vi "Actor Core.vi"(8 "error in":errorcluster, 11 "Air Cooler Application":refnum<class "Air Cooler Application.lvclass">) -> (0 "error out":errorcluster, 3 "Actor out":refnum<class "Actor.lvclass">)   [LabVIEW 2025, in "Air Cooler Application.lvlib" / "Air Cooler Application.lvclass"]
doc: "This is Actor Core.vi, the main message handling loop for Actors. An actor usually just sits in this loop and processes messages as they arrive. Any error returned by the message Do.vi call will stop the loop, with error code 43 as the canonical signal to stop with no error sent to caller. Descendants may override that in Handle Error.vi."
uses:
  Air Cooler Application.lvclass
  C:/Program Files/National Instruments/LabVIEW 2025/vi.lib/ActorFramework/Actor/Actor.lvclass
  <vilib>/ActorFramework/Actor/Actor.lvclass
  Cooler/Cooler/Cooler.lvclass
  Live User Controller/Live User Controller.lvclass
  C:/Program Files/National Instruments/LabVIEW 2025/ProjectTemplates/Source/Core/Feedback Evaporative Cooler/Cooler Controller/Cooler Controller/Cooler Controller.lvclass
  <vilib>/ActorFramework/Actor/Actor.lvclass/Actor.ctl
  <vilib>/ActorFramework/Message Enqueuer/Message Enqueuer.lvclass/Message Enqueuer.ctl
  Air Cooler Application.lvclass/Air Cooler Application.ctl
  <vilib>/ActorFramework/Stop Msg/Stop Msg.lvclass/Stop Msg.ctl
  Programmatic Controller/Programmatic Controller.lvclass
  Swap Controllers Msg/Swap Controllers Msg.lvclass/Swap Controllers Msg.ctl
  Cooler Controller/Write Cooler Enqueuer Msg/Write Cooler Enqueuer Msg.lvclass/Write Cooler Enqueuer Msg.ctl
  Cooler/Write Controller Enqueuer Msg/Write Controller Enqueuer Msg.lvclass/Write Controller Enqueuer Msg.ctl
  <vilib>/ActorFramework/Message Enqueuer/Init from Existing Queue.vi
  <vilib>/ActorFramework/Message Enqueuer/Enqueue.vi
  <vilib>/ActorFramework/Message Enqueuer/Enqueue Critical.vi
  Cooler Controller/Write Cooler Enqueuer Msg/Write Cooler Enqueuer Msg.lvclass
  C:/Program Files/National Instruments/LabVIEW 2025/vi.lib/ActorFramework/Message/Message.lvclass
  Cooler/Write Controller Enqueuer Msg/Write Controller Enqueuer Msg.lvclass
  <vilib>/ActorFramework/Stop Msg/Stop Msg.lvclass
  Swap Controllers Msg/Swap Controllers Msg.lvclass
  <vilib>/ActorFramework/Message Priority Queue/Priority Enqueue.vi
  <vilib>/ActorFramework/Message Enqueuer/Message Enqueuer.lvclass
panel:
  in  "DNL_Controller Selection":enum32{"UI Option 1", "UI Option 2"}(radio)
  in  "Stop":bool
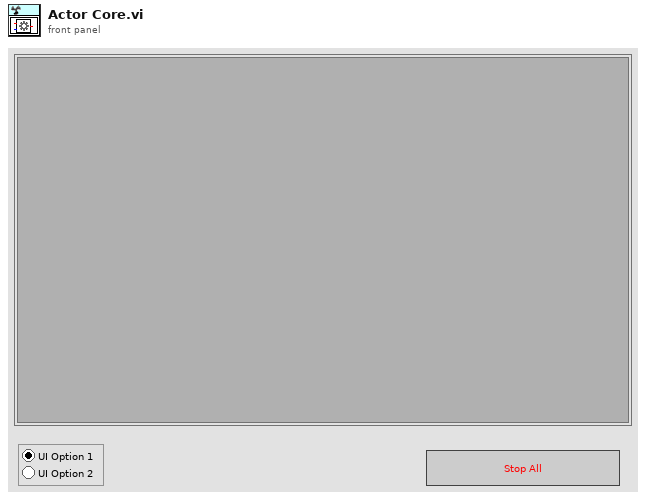
[diagram p1: front panel]
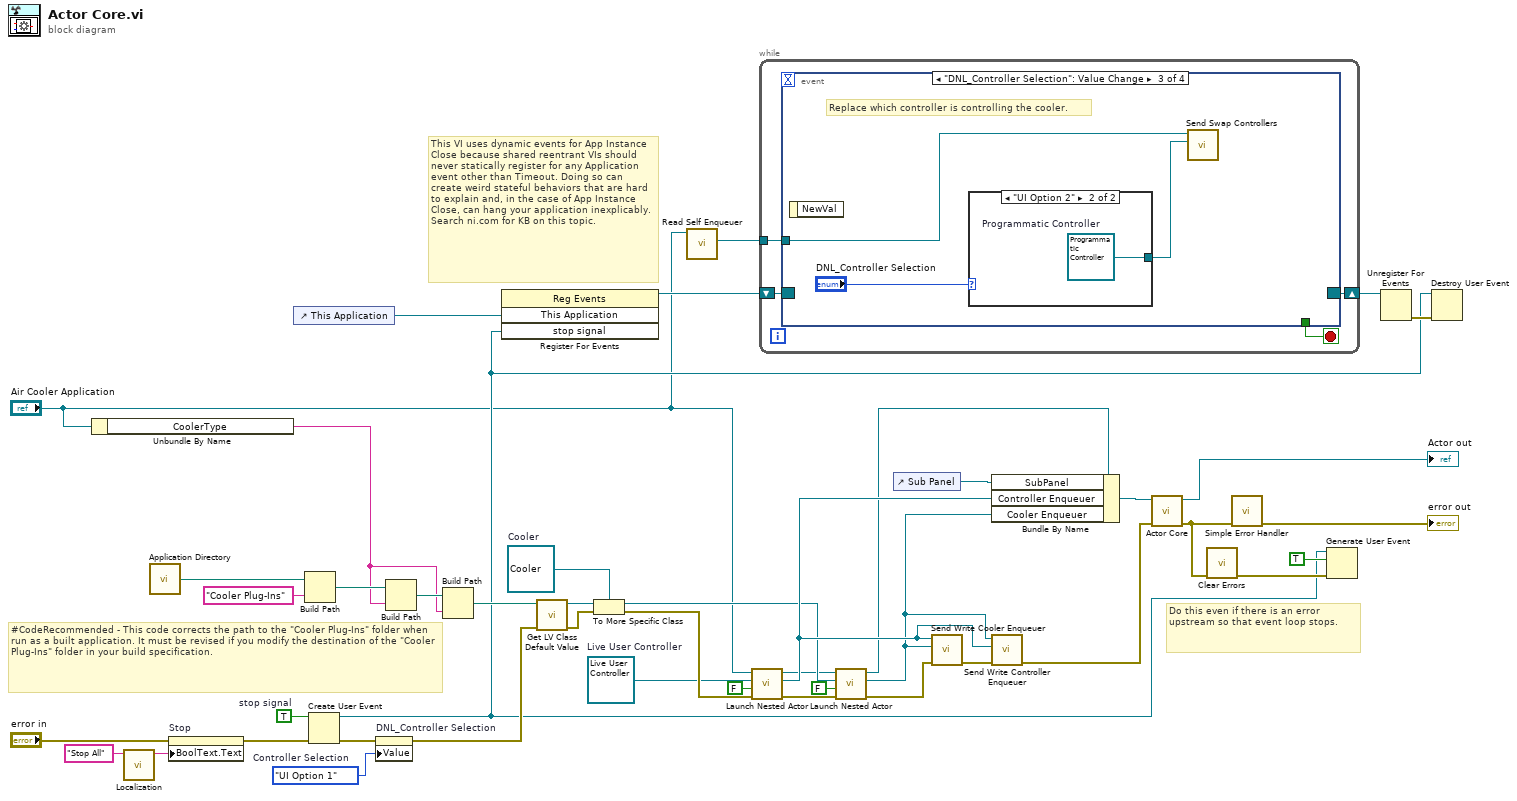
[diagram p0: block diagram]
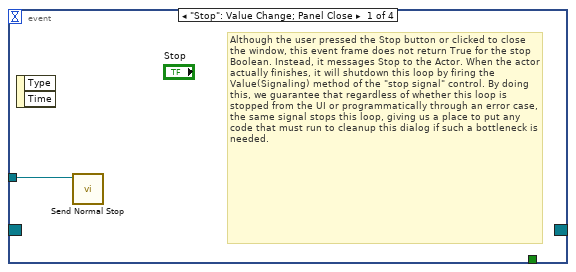
[diagram p2: hidden frame]
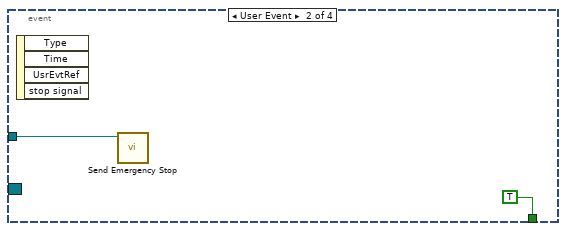
[diagram p3: hidden frame]
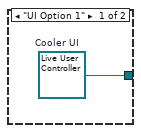
[diagram p4: hidden frame]
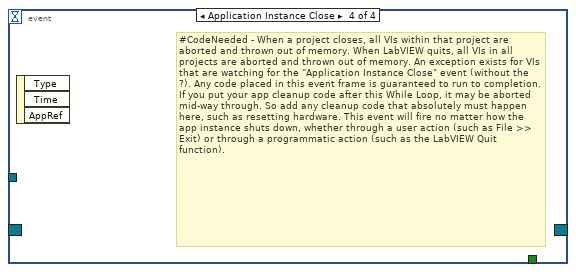
[diagram p5: hidden frame]
diagram:
  w9 = enum32{"UI Option 1", "UI Option 2"}."UI Option 1"  # Controller Selection
  w22 = TRUE  # stop signal
  w6 = refnum<class "Live User Controller.lvclass"> refnum  # Live User Controller
  w34 = refnum<class "Cooler.lvclass"> refnum  # Cooler
  # "This VI uses dynamic events for App Instance Close because shared reentrant VIs should never statically register for any Application event other than Timeout. Doing so can create weird stateful behaviors that are hard to explain and, in the case of App Instance Close, can hang your application inexplicably. Search ni.com for KB on this topic."
  # "#CodeRecommended - This code corrects the path to the \"Cooler Plug-Ins\" folder when run as a built application. It must be revised if you modify the destination of the \"Cooler Plug-Ins\" folder in your build specification."
  # "Do this even if there is an error upstream so that event loop stops."
  n1 = Unbundle By Name("Air Cooler Application") -> ("CoolerType"=w27:string)
  n2 = call "Localization.vi"("Unlocalized"="Stop All") -> ("Localized"=w39:string)  [unwired: 10 in]
  n3 = call <vilib>:"Application Directory.vi"() -> ("Application Directory"=w10:path)
  n4 = property on="Stop" class="Bool"(error in="error in", "BoolText.Text"=w39) -> (error out=w23:errorcluster)  [unwired: 1 in, 1 out]
  n5 = control-ref of="This Application"() -> (w11:refnum<vi>)
  n6 = Build Path(base path=w10, name or relative path="Cooler Plug-Ins") -> (appended path=w30:path)
  n7 = Create User Event(user event datatype=w22, error in=w23) -> (user event=w12:refnum<user-event>, error out=w16:errorcluster)
  n8 = property on="DNL_Controller Selection" class="RadioBtnsControl (strict)"(error in=w16, "Value"=w9) -> (error out=w15:errorcluster)  [unwired: 1 in, 1 out]
  n9 = Build Path(base path=w30, name or relative path=w27) -> (appended path=w38:path)
  n10 = Build Path(base path=w38, name or relative path=w27) -> (appended path=w37:path)
  n11 = register-events(w11, w12) -> (reference out=w21:refnum<event-registration>)  [unwired: 2 in, 1 out]
  n12 = call <vilib>:"Get LV Class Default Value.vi"("error in (no error)"=w15, "class path"=w37) -> ("error out"=w35:errorcluster, "object"=w36:refnum<class>)  [unwired: 8 in]
  n13 = To More Specific Class(target class=w34, reference=w36, error in=w35) -> (specific class reference=w8:refnum<class "Cooler.lvclass">, error out=w26:errorcluster)
  n14 = call <vilib>:"Read Self Enqueuer.vi"("Actor"="Air Cooler Application") -> ("Self Enqueuer"=w7:refnum<class "Message Enqueuer.lvclass">)  [unwired: 10 in]
  n15 = call <vilib>:"Launch Nested Actor.vi"("error in (no error)"=w26, "Auto-stop? (T)"=FALSE, "Nested Actor"=w6, "Caller Actor in"="Air Cooler Application") -> ("error out"=w43:errorcluster, "Nested Actor's Enqueuer"=w25:refnum<class "Message Enqueuer.lvclass">, "Caller Actor out"=w5:refnum<class "Air Cooler Application.lvclass">)  [unwired: 5 in]
  n16 = while {
    tunnel: w7 -> [w48]
    shift-right: [w45] -> w18
    shift-left: w21 -> [w46]
    stop <- w47 stop-if-true
    n17 = event shown="[2] \"DNL_Controller Selection\": Value Change" {
      selector: w46 -> [_ _ _ _]
      dyn-events: [_ _ _ _] -> w45
      timeout: _ -> [_ _ _ _]
      tunnel: w48 -> [w49 w51 w54 _]
      tunnel: [_ TRUE _ _] -> w47
      event "Stop": Value Change; Panel Close {
        # "Although the user pressed the Stop button or clicked to close the window, this event frame does not return True for the stop Boolean. Instead, it messages Stop to the Actor. When the actor actually finishes, it will shutdown this loop by firing the Value(Signaling) method of the \"stop signal\" control. By doing this, we guarantee that regardless of whether this loop is stopped from the UI or programmatically through an error case, the same signal stops this loop, giving us a place to put any code that must run to cleanup this dialog if such a bottleneck is needed."
        n18 = event-data() -> ()  [unwired: 1 in, 2 out]
        n19 = call <vilib>:"Send Normal Stop.vi"("Message Enqueuer"=w49) -> ()  [unwired: 10 in, 1 out]
      }
      event User Event {
        n20 = event-data() -> ()  [unwired: 1 in, 4 out]
        n21 = call <vilib>:"Send Emergency Stop.vi"("Message Enqueuer"=w51) -> ()  [unwired: 10 in, 1 out]
      }
      event "DNL_Controller Selection": Value Change {
        # "Replace which controller is controlling the cooler."
        n22 = event-data() -> ()  [unwired: 1 in, 1 out]
        n23 = case shown="\"UI Option 2\"" "DNL_Controller Selection" {
          tunnel: [w55 w56] -> w52
          frame "UI Option 1" {
            w55 = refnum<class "Live User Controller.lvclass"> refnum  # Cooler UI
          }
          frame "UI Option 2" {
            w56 = refnum<class "Programmatic Controller.lvclass"> refnum  # Programmatic Controller
          }
        }
        n24 = call "Send Swap Controllers.vi"("Cooler Controller"=w52, "Message Enqueuer"=w54) -> ()  [unwired: 9 in, 1 out]
      }
      event Application Instance Close {
        # "#CodeNeeded - When a project closes, all VIs within that project are aborted and thrown out of memory. When LabVIEW quits, all VIs in all projects are aborted and thrown out of memory. An exception exists for VIs that are watching for the \"Application Instance Close\" event (without the ?). Any code placed in this event frame is guaranteed to run to completion. If you put your app cleanup code after this While Loop, it may be aborted mid-way through. So add any cleanup code that absolutely must happen here, such as resetting hardware. This event will fire no matter how the app instance shuts down, whether through a user action (such as File >> Exit) or through a programmatic action (such as the LabVIEW Quit function)."
        n25 = event-data() -> ()  [unwired: 1 in, 3 out]
      }
    }
  }
  n26 = call <vilib>:"Launch Nested Actor.vi"("error in (no error)"=w43, "Auto-stop? (T)"=FALSE, "Nested Actor"=w8, "Caller Actor in"=w5) -> ("error out"=w32:errorcluster, "Nested Actor's Enqueuer"=w24:refnum<class "Message Enqueuer.lvclass">, "Caller Actor out"=w3:refnum<class "Air Cooler Application.lvclass">)  [unwired: 5 in]
  n27 = control-ref of="Sub Panel"() -> (w33:refnum<vi>)
  n28 = call "Send Write Cooler Enqueuer.vi"("error in (no error)"=w32, "Cooler Enqueuer"=w24, "Message Enqueuer"=w25) -> ("error out"=w29:errorcluster)  [unwired: 8 in]
  n29 = Bundle By Name(cluster=w3, "SubPanel"=w33, "Controller Enqueuer"=w25, "Cooler Enqueuer"=w24) -> (w42:refnum<class "Air Cooler Application.lvclass">)
  n30 = call "Send Write Controller Enqueuer.vi"("error in (no error)"=w29, "Controller Enqueuer"=w25, "Message Enqueuer"=w24) -> ("error out"=w28:errorcluster)  [unwired: 8 in]
  n31 = call-parent "Actor Core.vi"("error in"=w28, "Actor in"=w42) -> ("error out"=w14:errorcluster, "Actor out"=→"Actor out":refnum<class "Actor.lvclass">)  [unwired: 8 in]
  n32 = call <vilib>:"Clear Errors.vi"("error in (no error)"=w14) -> ("error out"=w20:errorcluster)  [unwired: 5 in, 1 out]
  n33 = call <vilib>:"Simple Error Handler.vi"("error in (no error)"=w14) -> ("error out"=→"error out":errorcluster)  [unwired: 4 in, 4 out]
  n34 = Generate User Event(user event=w12, event data cluster=TRUE ("stop"), error in=w20) -> ()  [unwired: 1 in, 2 out]
  n35 = Unregister For Events(event registration refnum=w18) -> (error out=w17:errorcluster)  [unwired: 1 in]
  n36 = Destroy User Event(user event=w12, error in=w17) -> ()  [unwired: 1 out]
